vi "Pre-Build Action.vi"(6 "Top Level/Always Included VIs":path[](array[path]), 7 "Main Destination Path":path, 9 "Target Name":string, 10 "Build Specification Name":string, 11 "Project Path":path) -> (0 "error out":errorcluster)   [LabVIEW 2020]
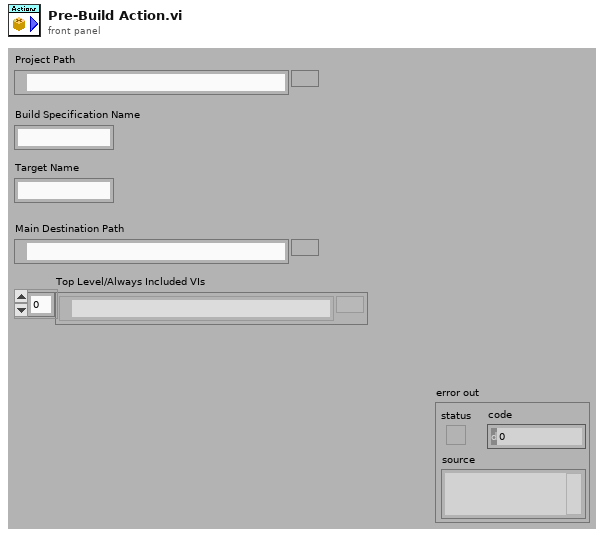
[diagram p1: front panel]
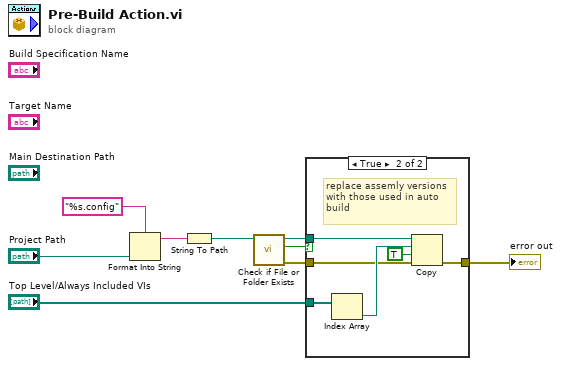
[diagram p0: block diagram]
diagram:
  n1 = Format Into String(format string="%s.config", "Project Path") -> (resulting string=w7:string)  [unwired: 2 in, 1 out]
  n2 = String To Path(string=w7) -> (path=w6:path)
  n3 = call <vilib>:"Check if File or Folder Exists.vi"("path"=w6) -> ("error out"=w2:errorcluster, "file or folder exists?"=w4:bool, "dup path"=w5:path)  [unwired: 8 in]
  n4 = case shown="True" w4 {
    tunnel: w5 -> [_ w15]
    tunnel: "Top Level/Always Included VIs" -> [_ w16]
    tunnel: w2 -> [w10 w13]
    tunnel: [w10 w11] -> w1
    frame False {
    }
    frame True {
      # "replace assemly versions\nwith those used in auto\nbuild"
      n5 = Index Array(array=w16) -> (element=w14:path)  [unwired: 1 in]
      n6 = Copy(8:w13, 9:TRUE ("overwrite (F)"), 10:w14, 11:w15) -> (0:w11:errorcluster)  [unwired: 1 in, 2 out]
    }
  }
  "error out" <- w1
